vi "Update Datatypes Enum.vi"() -> ()   [LabVIEW 2015, in "Modbus Module editor node.lvclass"]
uses:
  Modbus Module editor node.lvclass
  <vilib>/NI/Tag Bus/tag/Data Type.ctl
  <vilib>/NI/Tag Bus/tag/tag descriptor.lvclass
panel:
  in  "Data Type":T1
  in  "supported types":T1[](array[typedef])=[enum."Double", enum."Single", enum."I64", enum."I32", enum."I16", enum."I8", enum."U64", enum."U32", enum."U16", enum."U8", enum."Boolean", enum."String"]
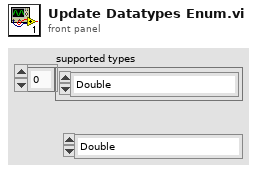
[diagram p1: front panel]
types:
  T1 = typedef "tag bus.lvlib/tag descriptor.lvclass/Data Type.ctl" = enum16{"Double", "Single", "I64", "I32", "I16", "I8", "U64", "U32", "U16", "U8", "Boolean", "String", "Array of Double", "Array of Single", "Array of I64", "Array of I32", "Array of I16", "Array of I8", "Array of U64", "Array of U32", "Array of U16", "Array of U8", "Array of Boolean", "Array of String"}
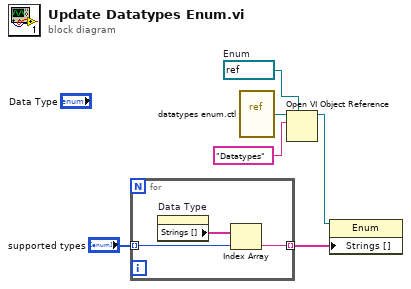
[diagram p0: block diagram]
diagram:
  w4 = refnum<vi> refnum  # Enum
  n1 = for {
    tunnel: "supported types" -> [w8] mode=indexing
    tunnel: [w7] -> w1 mode=indexing
    n2 = property on="Data Type" class="Enum (strict)"() -> ("Strings []"=w9:string[])  [unwired: 2 in, 2 out]
    n3 = Index Array(array=w9, index=w8) -> (element=w7:string)
  }
  n4 = vi-ref "datatypes enum.ctl"() -> (w6:refnum<vi>)
  n5 = Open VI Object Reference(7:w4, 10:"Datatypes" ("name/order"), 11:w6) -> (3:w3:refnum<vi>)  [unwired: 1 in, 1 out]
  n6 = property class="Enum"(reference=w3, "Strings []"=w1) -> ()  [unwired: 1 in, 2 out]
